vi "Calc_R.vi"(11 "Radius":dbl) -> (3 "V (km/s)":dbl)   [LabVIEW 2012]
panel:
  out "Platescale (rad)":dbl=3.4
  out "Platescale (arcsec)":dbl=3.4
  in  "n_ref":dbl=3.4
  out "dV (km/s)":dbl
  out "R":dbl
  out "1/R":dbl
  in  "Width":dbl
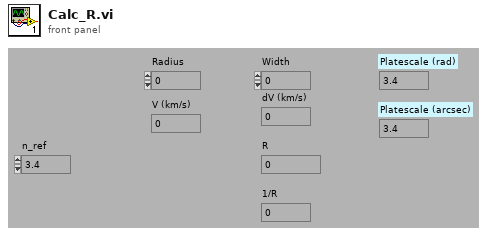
[diagram p1: front panel]
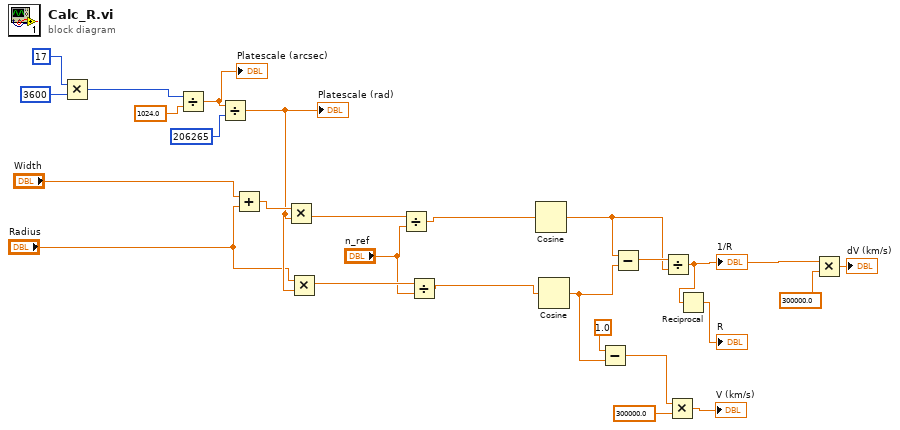
[diagram p0: block diagram]
diagram:
  n1 = Multiply(x=17, y=3600) -> (x*y=w24:i32)
  n2 = Divide(x=w24, y=1024.0) -> (x/y=w3:dbl)
  "Platescale (arcsec)" <- w3
  n3 = Divide(x=w3, y=206265) -> (x/y=w2:dbl)
  "Platescale (rad)" <- w2
  n4 = Add(x="Width", y="Radius") -> (x+y=w23:dbl)
  n5 = Multiply(x=w23, y=w2) -> (x*y=w13:dbl)
  n6 = Multiply(x="Radius", y=w2) -> (x*y=w11:dbl)
  n7 = Divide(x=w13, y="n_ref") -> (x/y=w12:dbl)
  n8 = Divide(x=w11, y="n_ref") -> (x/y=w9:dbl)
  n9 = Cosine(x=w12) -> (cos(x)=w21:dbl)
  n10 = Cosine(x=w9) -> (cos(x)=w5:dbl)
  n11 = Subtract(x=1.0 ("y"), y=w5) -> (x-y=w4:dbl)
  n12 = Subtract(x=w21, y=w5) -> (x-y=w22:dbl)
  n13 = Divide(x=w22, y=w21) -> (x/y=w19:dbl)
  "1/R" <- w19
  n14 = Multiply(x=w4, y=300000.0) -> (x*y=→"V (km/s)":dbl)
  n15 = Reciprocal(x=w19) -> (1/x=→"R":dbl)
  n16 = Multiply(x=w19, y=300000.0) -> (x*y=→"dV (km/s)":dbl)
